vi "Config PDC Framed Timeslot.vi"(0 "VISA Resource Name":refnum<visa-resource-name>, 1 "Data (0:PN9)":T1(ring), 2 "FIX4 (0000)":i16 format="%.0b", 3 "User File Name (BIN_DATA)":string="BIN_DATA", 5 "Timeslot (0)":i16, 7 "Status (T:ON)":bool=TRUE, 9 "Timeslot Type (2:UP TCH)":T2(ring)=enum."UP TCH", 11 "error in (no error)":errorcluster {"code" format="%.0x"}, 12 "SYNC (785B4)":i32=492980 format="%.0x", 13 "SACCH (0000)":i32 format="%.0x", 14 "CC (00)":i32 format="%.0x") -> (4 "VISA Resource Name Out":refnum<visa-resource-name>, 15 "error out":errorcluster {"code" format="%.0x"})   [LabVIEW 2012, in "Agilent ESG Series.lvlib"]
doc: "This VI is used configure a specified Timeslot.\nRun the Config PDC Framed.vi before running this vi.\nRun this vi multiple times to configure multiple Timeslots."
uses:
  <instrlib>/Agilent ESG Series/Agilent ESG Series.lvlib
panel:
  # "ON"
  # "OFF"
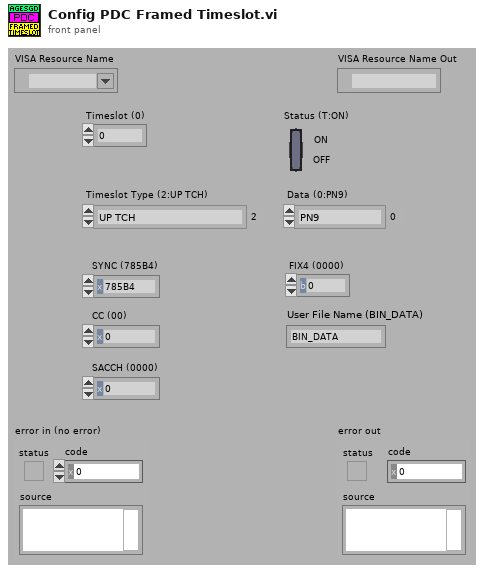
[diagram p1: front panel]
types:
  T1 = enum16{"PN9", "PN15", "FIX4", "USER FILE", "EXT", "4 1's & 4 0's", "8 1's & 8 0's", "16 1's & 16 0's", "32 1's & 32 0's", "64 1's & 64 0's"}
  T2 = enum16{"UP CUSTOM", "DOWN CUSTOM", "UP TCH", "DOWN TCH", "UP VOX", "UP TCH ALL", "DOWN TCH ALL"}
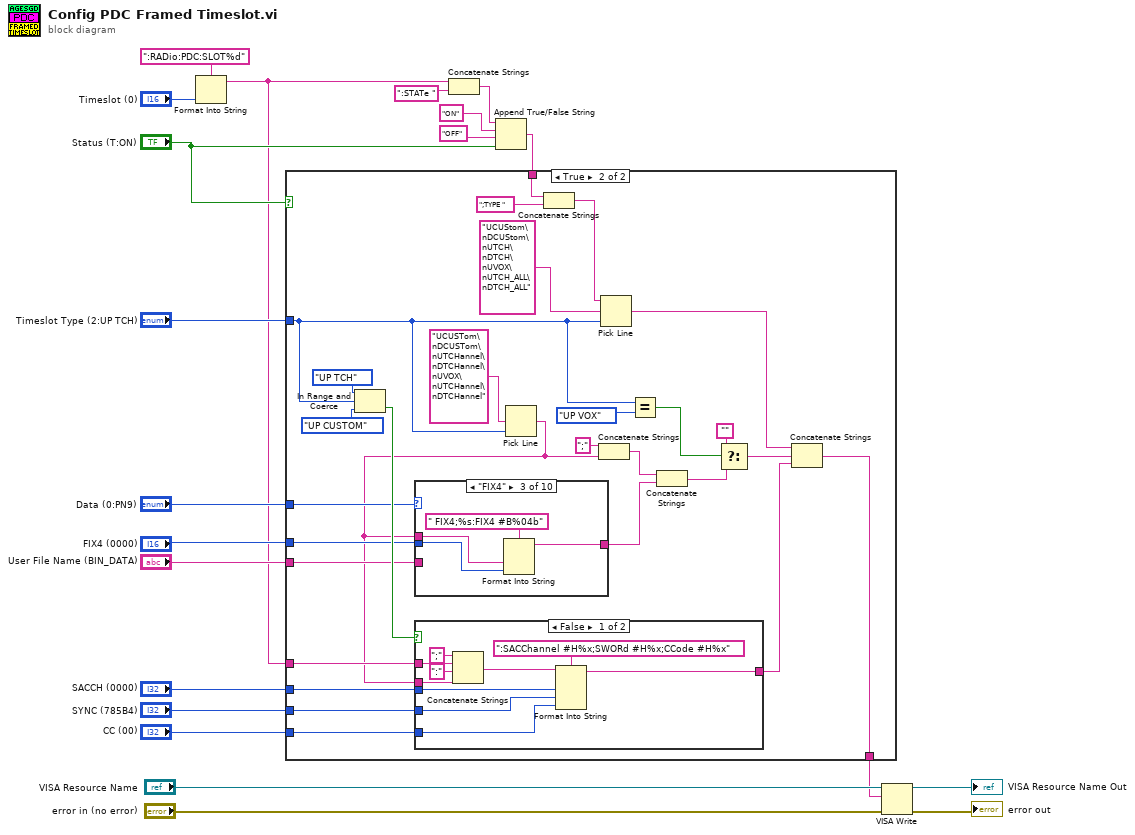
[diagram p0: block diagram]
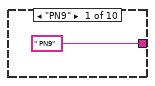
[diagram p3: hidden frame]
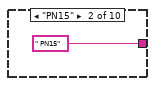
[diagram p4: hidden frame]
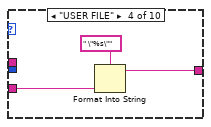
[diagram p5: hidden frame]
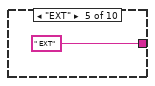
[diagram p6: hidden frame]
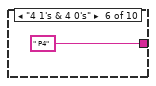
[diagram p7: hidden frame]
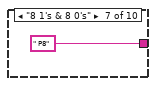
[diagram p8: hidden frame]
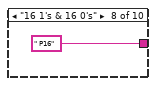
[diagram p9: hidden frame]
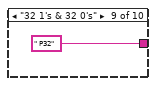
[diagram p10: hidden frame]
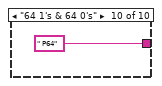
[diagram p11: hidden frame]
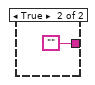
[diagram p12: hidden frame]
diagram:
  n1 = Format Into String(format string=":RADio:PDC:SLOT%d", "Timeslot (0)") -> (resulting string=w3:string)  [unwired: 2 in, 1 out]
  n2 = Concatenate Strings(w3, ":STATe ") -> (w13:string)
  n3 = Append True/False String(1:"Status (T:ON)", 2:"OFF" ("false string"), 3:"ON" ("true string"), 4:w13) -> (0:w12:string)
  n4 = case shown="True" "Status (T:ON)" {
    tunnel: [w22 w50] -> w1
    tunnel: "Timeslot Type (2:UP TCH)" -> [_ w25]
    tunnel: "CC (00)" -> [_ w49]
    tunnel: "SYNC (785B4)" -> [_ w48]
    tunnel: "SACCH (0000)" -> [_ w47]
    tunnel: "FIX4 (0000)" -> [_ w43]
    tunnel: "User File Name (BIN_DATA)" -> [_ w42]
    tunnel: "Data (0:PN9)" -> [_ w41]
    tunnel: w12 -> [w22 w40]
    tunnel: w3 -> [_ w36]
    frame False {
    }
    frame True {
      n5 = In Range and Coerce(upper limit=T2."UP TCH" ("hi"), x=w25, lower limit=T2."UP CUSTOM" ("lo")) -> (In Range?=w45:bool)  [unwired: 1 out]
      n6 = Pick Line(multi-line string="UCUSTom\nDCUSTom\nUTCHannel\nDTCHannel\nUVOX\nUTCHannel\nDTCHannel", line index=w25) -> (output string=w30:string)  [unwired: 1 in]
      n7 = case shown="\"FIX4\"" w41 {
        tunnel: w42 -> [_ _ _ w59 _ _ _ _ _ _]
        tunnel: w43 -> [_ _ w54 _ _ _ _ _ _ _]
        tunnel: [" PN9" " PN15" w55 w57 " EXT" " P4" " P8" " P16" " P32" " P64"] -> w32
        tunnel: w30 -> [_ _ w53 _ _ _ _ _ _ _]
        frame "PN9" {
        }
        frame "PN15" {
        }
        frame "FIX4" {
          n8 = Format Into String(format string=" FIX4;%s:FIX4 #B%04b", w53, w54) -> (resulting string=w55:string)  [unwired: 2 in, 1 out]
        }
        frame "USER FILE" {
          n9 = Format Into String(format string=" \"%s\"", w59) -> (resulting string=w57:string)  [unwired: 2 in, 1 out]
        }
        frame "EXT" {
        }
        frame "4 1's & 4 0's" {
        }
        frame "8 1's & 8 0's" {
        }
        frame "16 1's & 16 0's" {
        }
        frame "32 1's & 32 0's" {
        }
        frame "64 1's & 64 0's" {
        }
      }
      n10 = case shown="False" w45 {
        tunnel: w47 -> [w75 _]
        tunnel: w48 -> [w74 _]
        tunnel: w49 -> [w73 _]
        tunnel: [w71 ""] -> w33
        tunnel: w36 -> [w70 _]
        tunnel: w30 -> [w67 _]
        frame False {
          n11 = Concatenate Strings(";", w70, ":" ("output string"), w67) -> (w69:string)
          n12 = Format Into String(format string=":SACChannel #H%x;SWORd #H%x;CCode #H%x", initial string=w69, w75, w74, w73) -> (resulting string=w71:string)  [unwired: 1 in, 1 out]
        }
        frame True {
        }
      }
      n13 = Concatenate Strings(w40, ";TYPE ") -> (w38:string)
      n14 = Concatenate Strings(";", w30) -> (w29:string)
      n15 = Pick Line(string ("")=w38, multi-line string="UCUStom\nDCUStom\nUTCH\nDTCH\nUVOX\nUTCH_ALL\nDTCH_ALL", line index=w25) -> (output string=w35:string)
      n16 = Equal?(x=w25, y=T2."UP VOX") -> (x = y?=w23:bool)
      n17 = Concatenate Strings(w29, w32) -> (w28:string)
      n18 = Select(t="", s=w23, f=w28) -> (s? t:f=w27:string)
      n19 = Concatenate Strings(w35, w27, w33) -> (w50:string)
    }
  }
  n20 = VISA Write(VISA resource name="VISA Resource Name", write buffer=w1, error in (no error)="error in (no error)") -> (VISA resource name out=→"VISA Resource Name Out":refnum<visa-resource-name>, error out=→"error out":errorcluster)  [unwired: 1 out]
